vi "_refreshChart_EEPROM_vna_wmg.vi"(0 "operKey":string="SFP+", 1 "refKey":string="SFP+", 2 "chart_step2 2":refnum<vi>, 3 "oper":enum16{"refresh", "insert"}(ring), 4 "insertArray":string[][](array[string])) -> ()   [LabVIEW 2011]
panel:
  out "子数组":string[][](array[string])
  out "输出数组":string[][](array[string])
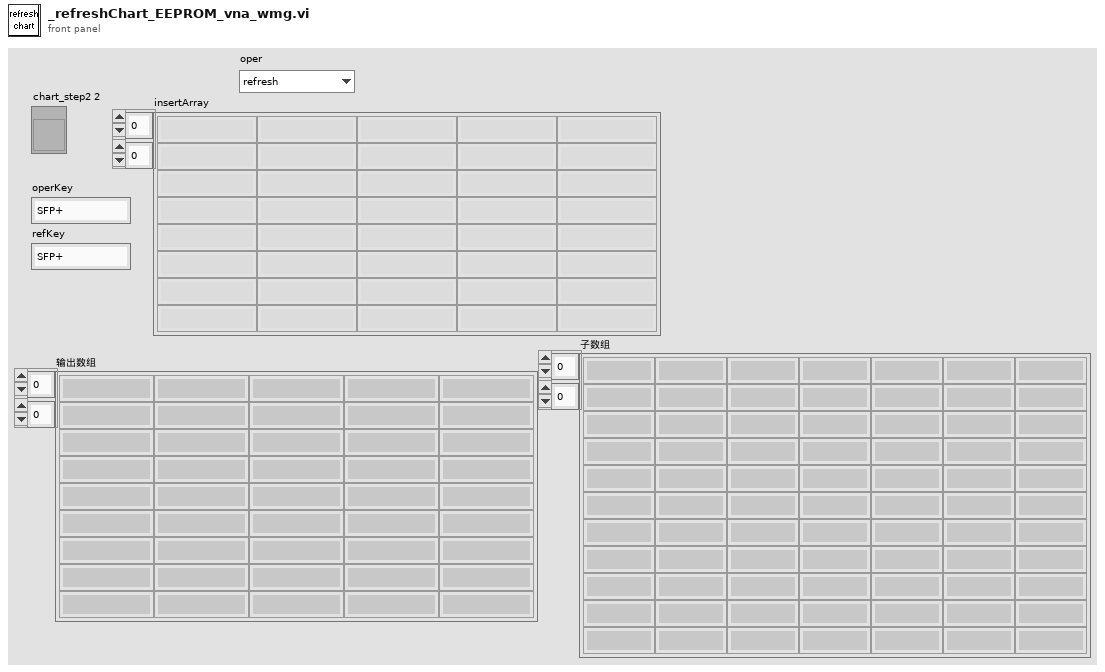
[diagram p1: front panel]
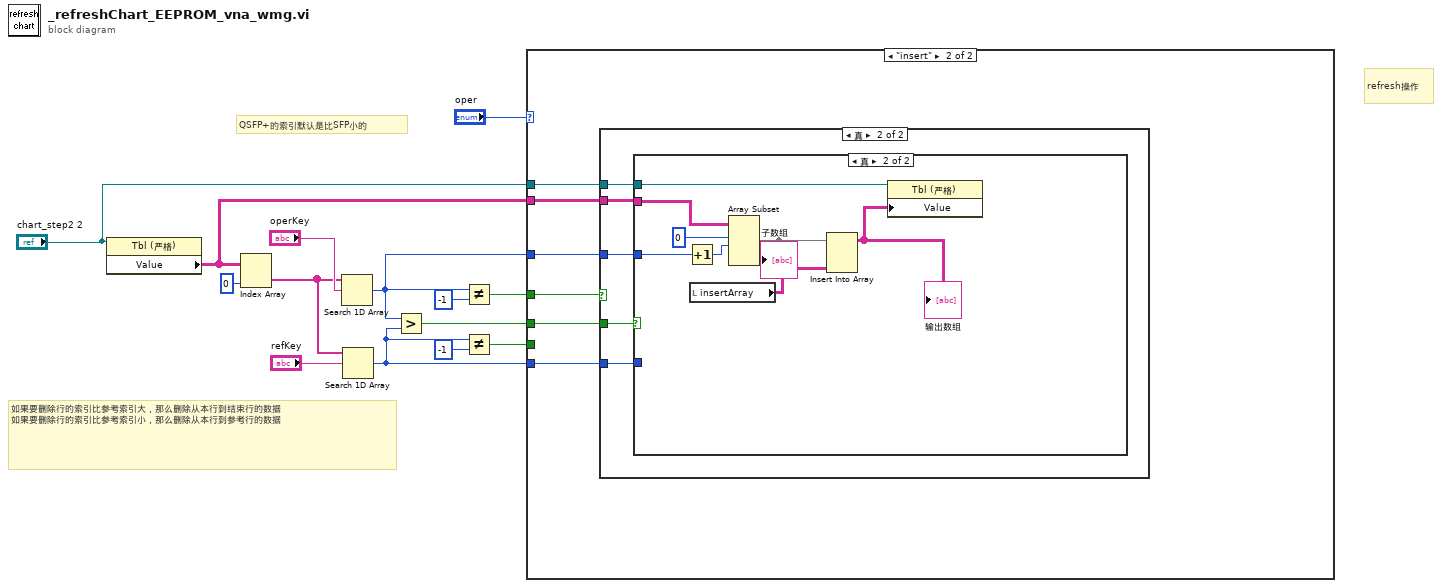
[diagram p0: block diagram]
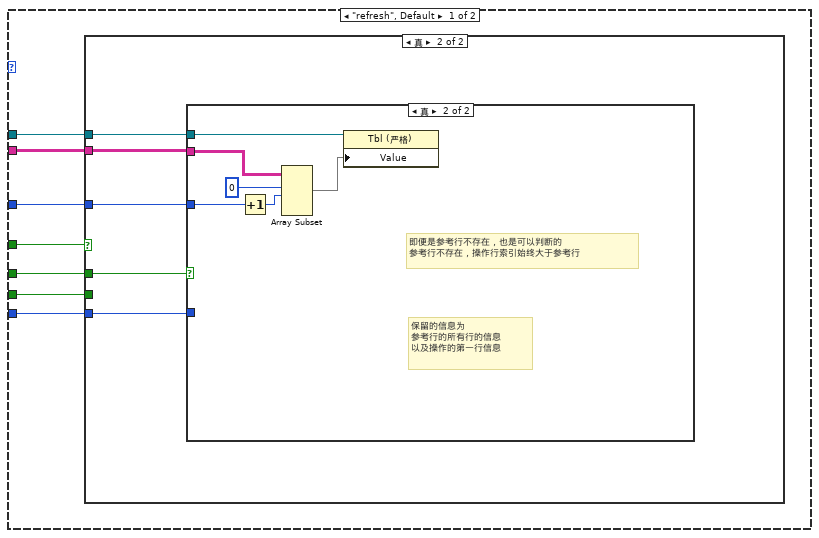
[diagram p2: hidden frame]
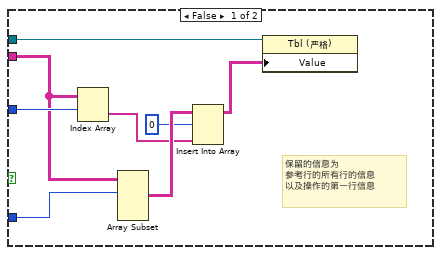
[diagram p4: hidden frame]
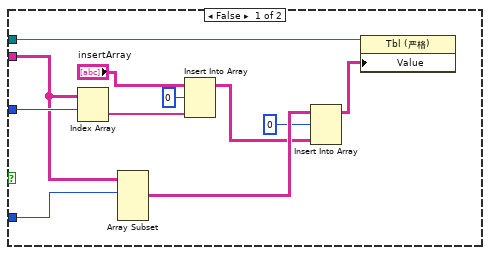
[diagram p6: hidden frame]
diagram:
  # "refresh操作"
  # "如果要删除行的索引比参考索引大，那么删除从本行到结束行的数据\n如果要删除行的索引比参考索引小，那么删除从本行到参考行的数据"
  # "QSFP+的索引默认是比SFP小的"
  n1 = property class="Tbl (严格)"(reference="chart_step2 2") -> ("Value"=w9:string[][])  [unwired: 1 in, 2 out]
  n2 = Index Array(array=w9, index (col)=0 ("禁用的索引 (列)")) -> (element=w11:string[])  [unwired: 1 in]
  n3 = Search 1D Array(1D array=w11, element="operKey") -> (index of element=w6:i32)  [unwired: 1 in]
  n4 = Search 1D Array(1D array=w11, element="refKey") -> (index of element=w2:i32)  [unwired: 1 in]
  n5 = Greater?(x=w6, y=w2) -> (0:w10:bool)
  n6 = Not Equal?(x=w6, y=-1) -> (x != y?=w4:bool)
  n7 = Not Equal?(x=w2, y=-1) -> (x != y?=w1:bool)
  n8 = case shown="\"insert\"" "oper" {
    tunnel: w10 -> [w21 w46]
    tunnel: w9 -> [w20 w45]
    tunnel: w6 -> [w19 w44]
    tunnel: "chart_step2 2" -> [w18 w43]
    tunnel: w2 -> [w17 w42]
    tunnel: w4 -> [w16 w41]
    tunnel: w1 -> [w15 _]
    frame "refresh", Default {
      n9 = case shown="真" w16 {
        tunnel: w21 -> [_ w26]
        tunnel: w20 -> [_ w25]
        tunnel: w19 -> [_ w24]
        tunnel: w18 -> [_ w23]
        tunnel: w17 -> [_ w22]
        tunnel: w15 -> [_ _]
        frame False {
        }
        frame True {
          n10 = case shown="真" w26 {
            tunnel: w23 -> [w27 w40]
            tunnel: w25 -> [w33 w36]
            tunnel: w24 -> [w34 w35]
            tunnel: w22 -> [w32 _]
            frame False {
              # "保留的信息为\n参考行的所有行的信息\n以及操作的第一行信息"
              n11 = Index Array(array=w33, index (row)=w34) -> (element=w30:string[])  [unwired: 1 in]
              n12 = Array Subset(array=w33, index (row)=w32) -> (w31:string[][])  [unwired: 3 in]
              n13 = Insert Into Array(array=w31, index (row)=0 ("索引 (行)"), new element=w30) -> (w28:string[][])  [unwired: 1 in]
              n14 = property class="Tbl (严格)"(reference=w27, "Value"=w28) -> ()  [unwired: 1 in, 2 out]
            }
            frame True {
              # "即便是参考行不存在，也是可以判断的\n参考行不存在，操作行索引始终大于参考行"
              # "保留的信息为\n参考行的所有行的信息\n以及操作的第一行信息"
              n15 = Increment(x=w35) -> (x+1=w39:i32)
              n16 = Array Subset(array=w36, index (row)=0 ("索引"), length (row)=w39) -> (w37:string[][])  [unwired: 2 in]
              n17 = property class="Tbl (严格)"(reference=w40, "Value"=w37) -> ()  [unwired: 1 in, 2 out]
            }
          }
        }
      }
    }
    frame "insert" {
      n18 = case shown="真" w41 {
        tunnel: w46 -> [_ w51]
        tunnel: w45 -> [_ w50]
        tunnel: w44 -> [_ w49]
        tunnel: w43 -> [_ w48]
        tunnel: w42 -> [_ w47]
        frame False {
        }
        frame True {
          n19 = case shown="真" w51 {
            tunnel: w48 -> [w56 w70]
            tunnel: w50 -> [w61 w67]
            tunnel: w49 -> [w62 w66]
            tunnel: w47 -> [w60 _]
            frame False {
              n20 = Index Array(array=w61, index (row)=w62) -> (element=w54:string[])  [unwired: 1 in]
              n21 = Array Subset(array=w61, index (row)=w60) -> (w59:string[][])  [unwired: 3 in]
              n22 = Insert Into Array(array="insertArray", index (row)=0 ("索引 (行)"), new element=w54) -> (w52:string[][])  [unwired: 1 in]
              n23 = Insert Into Array(array=w59, index (row)=0 ("索引 (行)"), new element=w52) -> (w57:string[][])  [unwired: 1 in]
              n24 = property class="Tbl (严格)"(reference=w56, "Value"=w57) -> ()  [unwired: 1 in, 2 out]
            }
            frame True {
              n25 = Increment(x=w66) -> (x+1=w69:i32)
              n26 = local read "insertArray"() -> (w64:string[][])
              n27 = Array Subset(array=w67, index (row)=0 ("索引"), length (row)=w69) -> (w65:string[][])  [unwired: 2 in]
              "子数组" <- w65
              n28 = Insert Into Array(array=w65, new element=w64) -> (w63:string[][])  [unwired: 2 in]
              "输出数组" <- w63
              n29 = property class="Tbl (严格)"(reference=w70, "Value"=w63) -> ()  [unwired: 1 in, 2 out]
            }
          }
        }
      }
    }
  }
